vi "CE Measure.vi"(11 "CEmeter settings":T7={"AC Source"={"AC Source type"=enum."Fluke 5XXX calibrator", "VISA"="", "Ref. clock (Hz)"=0.0, "status ref"=refnum}, "TWM pipe"="\\\\.\\pipe\\TWM:server", "Measurement status ref"=refnum, "TWM Status ref"=refnum, "Abort ref"=refnum, "DC meter"={"DC meter type"=enum."H/A/K 3458", "DC meter VISA"="", "NPLC"=10, "status ref"=refnum}, "Measurement properties"={"Measurement frequencies (Hz)"=[1000.0], "Sampling frequency (Hz)"=500000.0, "Signal amplitude (V)"=4.5, "AC-DC settle time (s)"=20.0, "Record length (multiples of period)"=[1000.0, 10000.0, 1000.0], "Measurement template file"=path "", "Row of START keyword"=1, "Row of STOP keyword"=0, "Calculate RMS from samples"=FALSE, "AC-DC warm up time (s)"=300.0, "Measurement template line"=[], "DC meter readings No."=10, "Algorithm"="TWM-WFFT"}, "Skip waiting ref"=refnum, "Octave paths"={"GNU Octave path"=path "C:/Program Files/GNU Octave/Octave-6.2.0/mingw64/bin", "TWM+QWTB path"=path "C:/Users/labina/Desktop/TWM-1.8.7.0-full/octprog", "lvlib path"=path "D:/martin/WAC/WACsw - github/control_software/Filter function meter/external libraries/GOLPI 0.7.3.1 source distribution LV 20.0 32 bit/lv_proc.dll"}, "Template definition"={"Keywords column"=0, "Sig. freq. column"=1, "Rec. len. column"=2, "Meas. points. row min to read"=9, "Meas. points. row max to read"=1509, "Properties column"=4, "Properties row start"=1, "Properties row end"=5, "Keyword START regexp"="", "Keyword STOP regexp"="", "HW data column"=7, "HW data row start"=1, "HW data row end"=3, "TIme and date column start"=3, "Digitizer value column start "=4, "DC mean column start "=6, "DC readings column start"=10}} {"Measurement properties"."Record length (multiples of period)" format="%#_3p"; "Measurement properties"."Sampling frequency (Hz)" format="%#_3p"; "Measurement properties"."Measurement frequencies (Hz)" format="%#_3p"}) -> (0 "error out":errorcluster)   [LabVIEW 2020]
uses:
  external libraries/varilib/varilib.lvlib
  external libraries/TWM-1.8.7.0-client/TWM Client.lvlib
  <vilib>/Utility/error.llb/DialogType.ctl
  Utilities/Type definitions/Sampling properties.ctl
  <vilib>/Utility/NIReport.llb/NI_report.lvclass
  General AC source/Type definitions/AC Source.ctl
  General AC source/Type definitions/AC Source type.ctl
  General DC meter/Type definitions/DC meter.ctl
  General DC meter/Type definitions/DC meter type.ctl
  FR Measurement/Type definitions/FR Measuement properties.ctl
  FR Utilities/Type definitions/FR Template definition.ctl
panel:
  out "TWM result as string for XCL":string[][][](array[string])
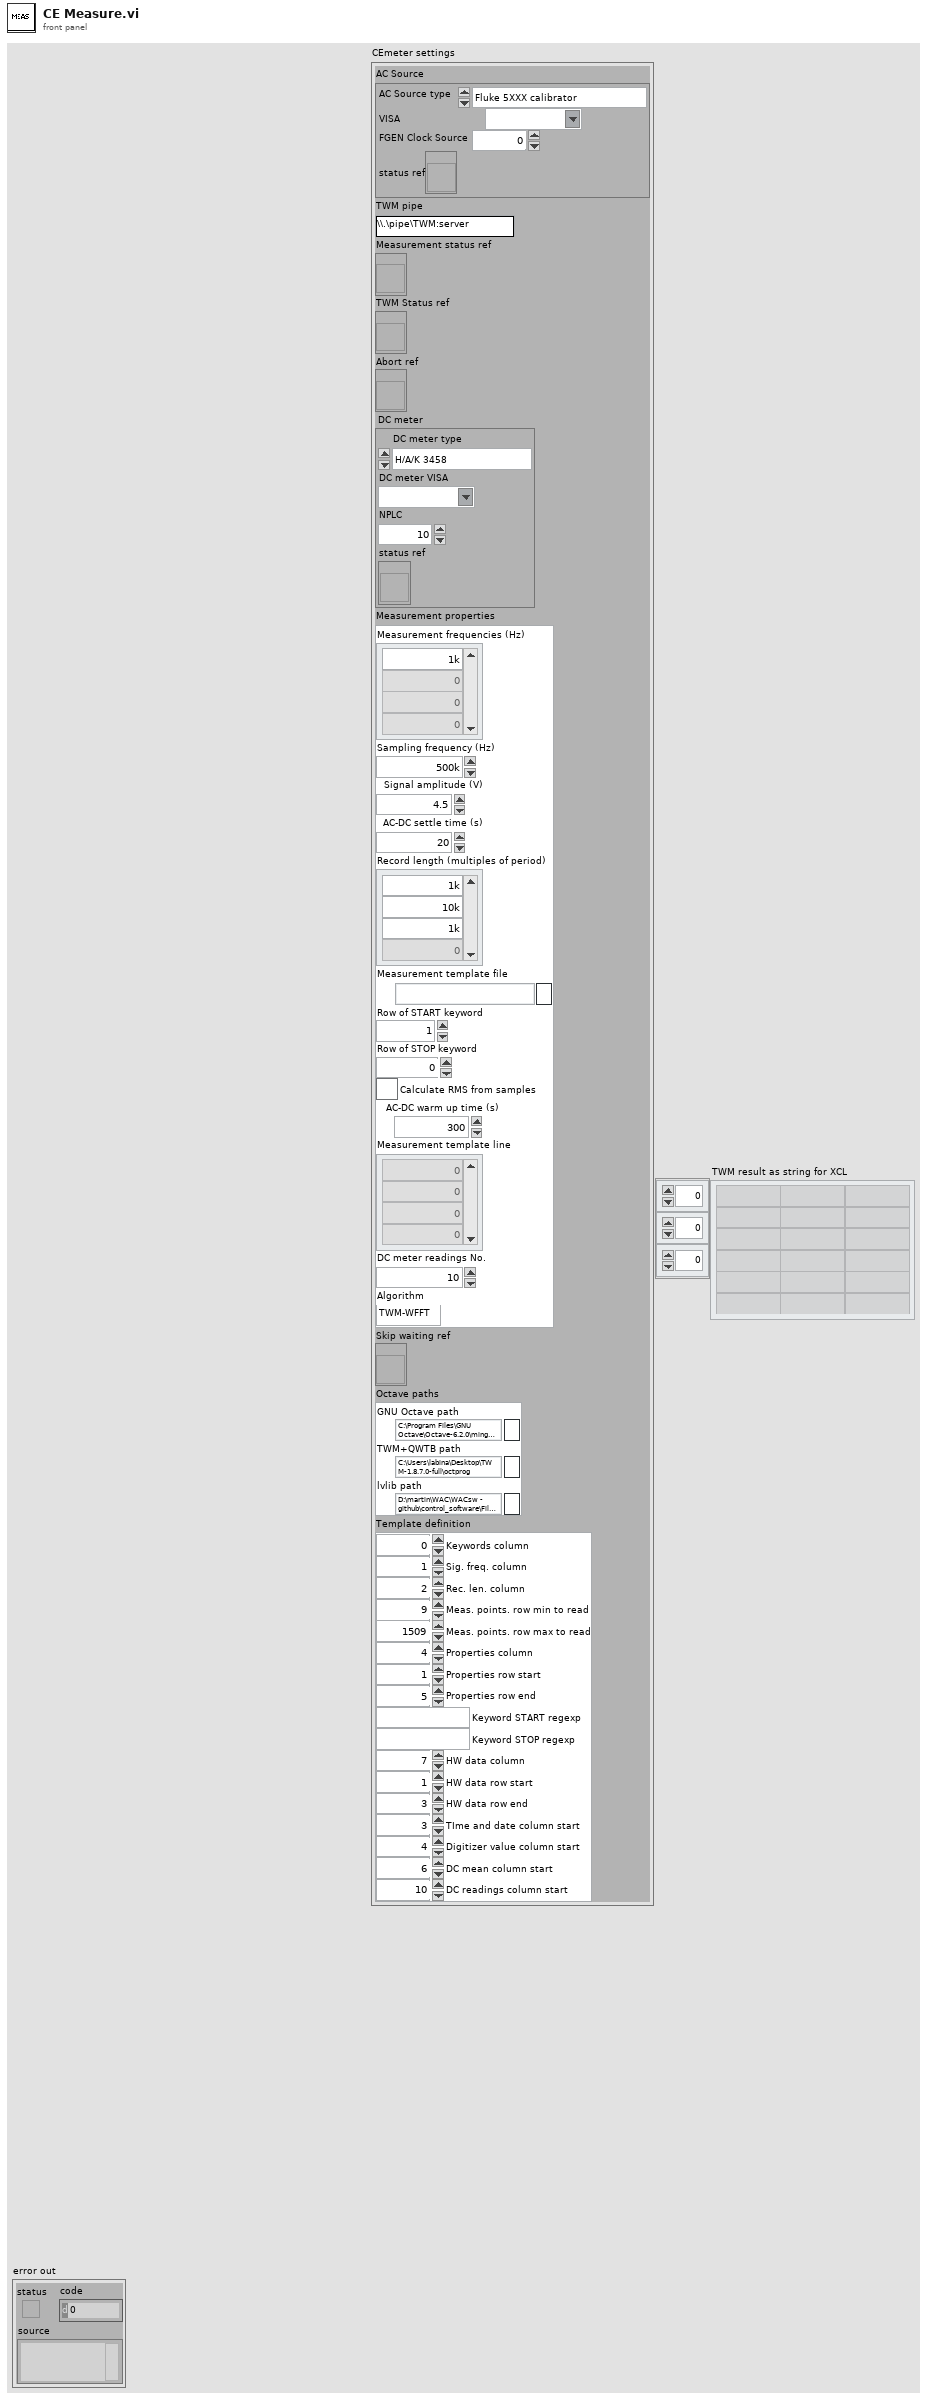
[diagram p1: front panel]
types:
  T1 = typedef "AC Source.ctl" = cluster{"AC Source type":T2, "VISA":refnum<visa-resource-name>, "Ref. clock (Hz)":dbl, "status ref":refnum<vi>}
  T2 = typedef "AC Source type.ctl" = enum16{"Fluke 5XXX calibrator", "Tektronix AFG3000 series", "dummy"}
  T3 = typedef "DC meter.ctl" = cluster{"DC meter type":T4, "DC meter VISA":refnum<visa-resource-name>, "NPLC":i32, "status ref":refnum<vi>}
  T4 = typedef "DC meter type.ctl" = enum16{"H/A/K 3458", "FLuke 8508A", "dummy"}
  T5 = typedef "FR Measuement properties.ctl" = cluster{"Measurement frequencies (Hz)":dbl[], "Sampling frequency (Hz)":dbl, "Signal amplitude (V)":dbl, "AC-DC settle time (s)":dbl, "Record length (multiples of period)":dbl[], "Measurement template file":path, "Row of START keyword":i32, "Row of STOP keyword":i32, "Calculate RMS from samples":bool, "AC-DC warm up time (s)":dbl, "Measurement template line":i32[], "DC meter readings No.":i32, "Algorithm":string}
  T6 = typedef "FR Template definition.ctl" = cluster{"Keywords column":i32, "Sig. freq. column":i32, "Rec. len. column":i32, "Meas. points. row min to read":i32, "Meas. points. row max to read":i32, "Properties column":i32, "Properties row start":i32, "Properties row end":i32, "Keyword START regexp":string, "Keyword STOP regexp":string, "HW data column":i32, "HW data row start":i32, "HW data row end":i32, "TIme and date column start":i32, "Digitizer value column start ":i32, "DC mean column start ":i32, "DC readings column start":i32}
  T7 = cluster{"AC Source":T1, "TWM pipe":string, "Measurement status ref":refnum<vi>, "TWM Status ref":refnum<vi>, "Abort ref":refnum<vi>, "DC meter":T3, "Measurement properties":T5, "Skip waiting ref":refnum<vi>, "Octave paths":cluster{"GNU Octave path":path, "TWM+QWTB path":path, "lvlib path":path}, "Template definition":T6}
  T8 = typedef "DialogType.ctl" = u16
  T9 = typedef "FFmeter settings.ctl" = cluster{"AC Source":T1, "TWM pipe":string, "Measurement status ref":refnum<vi>, "TWM Status ref":refnum<vi>, "Abort ref":refnum<vi>, "DC meter":T3, "Measurement properties":T5, "Skip waiting ref":refnum<vi>, "Octave paths":cluster{"GNU Octave path":path, "TWM+QWTB path":path, "lvlib path":path}, "Template definition":T6}
  T10 = typedef "Sampling properties.ctl" = cluster{"Sampling frequency (Hz)":dbl, "Record length (multiples of period)":dbl, "Signal amplitude (V)":dbl, "Measurement frequency (Hz)":dbl, "Calculate RMS from samples":bool, "Algorithm":string, "Measurement path":string}
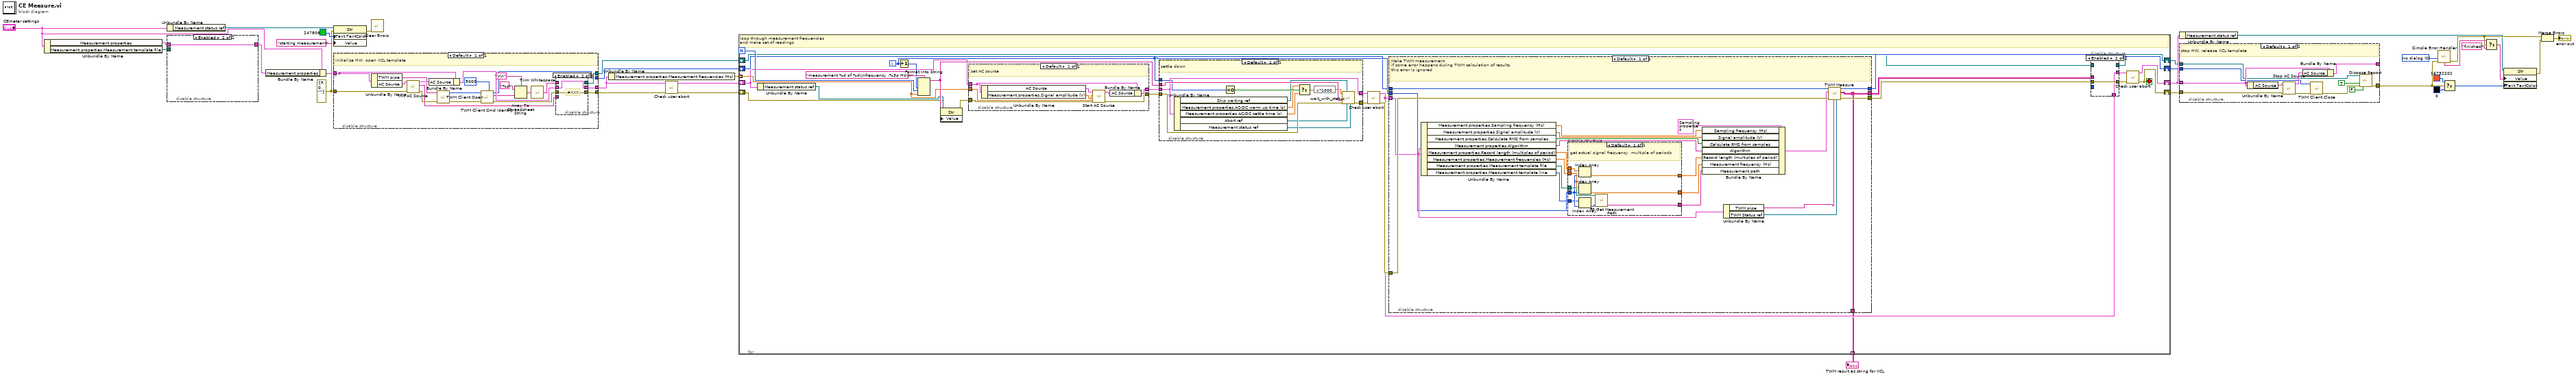
[diagram p0: block diagram]
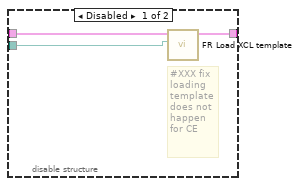
[diagram p2: hidden frame]
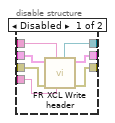
[diagram p3: hidden frame]
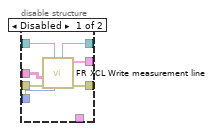
[diagram p4: hidden frame]
diagram:
  w30 = T8 0 items=["no dialog", "OK message", "continue or stop message", "OK message + warnings", "continue/stop + warnings"] ("type of dialog (OK msg:1)")
  w11 = errorcluster {"status"=FALSE, "code"=0, "source"=""} ("error out")
  n1 = Unbundle By Name("CEmeter settings") -> ("Measurement properties"=w9:T5, "Measurement properties.Measurement template file"=w5:path)
  n2 = Unbundle By Name("CEmeter settings") -> ("Measurement status ref"=w22:refnum<vi>)
  n3 = disable-structure shown="Enabled" {
    disable-tunnel: w9 -> [w37 w38]
    disable-tunnel: [w36 w38] -> w8
    disable-tunnel: w5 -> [w35 _]
    frame Disabled {
      # "#XXX fix\nloading\ntemplate\ndoes not\nhappen\nfor CE"
      n4 = call "FR Load XCL template.vi"("Measurement template file"=w35, "Measurement properties"=w37) -> ("Measurement properties out"=w36:T5)  [unwired: 9 in]
    }
    frame Enabled {
    }
  }
  n5 = Bundle By Name(cluster="CEmeter settings", "Measurement properties"=w8) -> (w6:T7)
  n6 = property class="Str"(reference=w22, error in=w11, "Text.TextColor"=u32 247808 ("Text.Text Colors:Text Color"), "Value"="starting measurement") -> (error out=w21:errorcluster)  [unwired: 1 out]
  n7 = disable-structure shown="Default" {
    disable-tunnel: w6 -> [w58]
    disable-tunnel: [w51] -> w2
    disable-tunnel: w11 -> [w56]
    disable-tunnel: [w54] -> w3
    disable-tunnel: [w43] -> w4
    disable-tunnel: [w52] -> w13
    frame Enabled {
      # "initialize HW, open XCL template"
      n8 = Unbundle By Name(w58) -> ("TWM pipe"=w55:string, "AC Source"=w59:T1)
      n9 = call "Init AC Source.vi"("error in (no error)"=w56, "AC source"=w59) -> ("error out"=w39:errorcluster, "Init status"=w50:string, "AC source out"=w57:T1)  [unwired: 7 in]
      n10 = Bundle By Name(cluster=w58, "AC Source"=w57) -> (w53:T7)
      n11 = call "TWM Client Open.vi"("error in"=w39, "pipe name"=w55) -> ("error out"=w45:errorcluster, "handle out"=w46:i32)  [unwired: 8 in]
      n12 = call "TWM Client Cmd Identify.vi"("timeout [ms]"=5000, "error in"=w45, "handle"=w46) -> ("error out"=w44:errorcluster, "channel idns"=w49:string[], "handle out"=w43:i32)  [unwired: 5 in, 1 out]
      n13 = Array To Spreadsheet String(delimiter (Tab)="\r\n", array=w49, 3:"%s" ("format string")) -> (spreadsheet string=w42:string)
      n14 = call <vilib>:"Trim Whitespace.vi"("string"=w42) -> ("trimmed string"=w41:string)  [unwired: 1 in]
      n15 = disable-structure shown="Enabled" {
        disable-tunnel: [w66 w67] -> w54
        disable-tunnel: w53 -> [w65 w68]
        disable-tunnel: [w64 _] -> w52
        disable-tunnel: [w63 w68] -> w51
        disable-tunnel: w50 -> [w62 _]
        disable-tunnel: w44 -> [w61 w67]
        disable-tunnel: w41 -> [w60 _]
        frame Disabled {
          n16 = call "FR XCL Write header.vi"("AC source idn"=w62, "Digitizer idn"=w60, "error in (no error)"=w61, "FFmeter settings"=w65) -> ("error out"=w66:errorcluster, "FFmeter settings out"=w63:T9, "NI_report out"=w64:refnum<class "NI_report.lvclass">)  [unwired: 5 in]
        }
        frame Enabled {
          # "#XXX"
        }
      }
    }
  }
  n17 = call <vilib>:"Clear Errors.vi"("error in (no error)"=w21) -> ()  [unwired: 5 in, 2 out]
  n18 = Unbundle By Name(w2) -> ("Measurement properties.Measurement frequencies (Hz)"=w34:dbl[])
  n19 = call "Check user abort.vi"("error in (no error)"=w3, "FFmeter settings"=w2) -> ("error out"=w20:errorcluster, "FFmeter settings out"=w19:T9)  [unwired: 8 in]
  n20 = for {
    N -> [w92]
    shift-right: [w82] -> w17
    shift-left: w20 -> [w86]
    shift-right: [w81] -> w15
    shift-left: w19 -> [w73]
    tunnel: w34 -> [w87] mode=indexing
    shift-right: [w77] -> w12
    shift-left: w13 -> [w76]
    shift-right: [w80] -> w14
    shift-left: w4 -> [w74]
    tunnel: [w69] -> w1 mode=indexing
    i -> [w72]
    stop <- w82 stop-if-true
    # "loop through measurement frequencies\nand make set of readings"
    n21 = Unbundle By Name(w73) -> ("Measurement status ref"=w91:refnum<vi>)
    n22 = Increment(x=w72) -> (x+1=w93:i32)
    n23 = Format Into String(format string="measurement %d of %d\\nfrequency :%3p Hz\\n", w93, w92, w87) -> (resulting string=w94:string)  [unwired: 2 in, 1 out]
    n24 = property class="Str"(reference=w91, error in=w86, "Value"=w94) -> (error out=w90:errorcluster)  [unwired: 1 out]
    n25 = disable-structure shown="Default" {
      disable-tunnel: w73 -> [w124]
      disable-tunnel: w90 -> [w123]
      disable-tunnel: [w122] -> w89
      disable-tunnel: [w125] -> w88
      disable-tunnel: w87 -> [w119]
      frame Enabled {
        # "set AC source"
        n26 = Unbundle By Name(w124) -> ("AC Source"=w120:T1, "Measurement properties.Signal amplitude (V)"=w118:dbl)
        n27 = call "Start AC Source.vi"("error in (no error)"=w123, "Signal amplitude (V)"=w118, "Signal frequency  (Hz)"=w119, "AC source"=w120) -> ("error out"=w122:errorcluster, "AC source out"=w121:T1)  [unwired: 5 in, 1 out]
        n28 = Bundle By Name(cluster=w124, "AC Source"=w121) -> (w125:T9)
      }
    }
    n29 = disable-structure shown="Default" {
      disable-tunnel: w94 -> [w117]
      disable-tunnel: [w111] -> w85
      disable-tunnel: [w115] -> w83
      disable-tunnel: w89 -> [w116]
      disable-tunnel: w88 -> [w115]
      disable-tunnel: w72 -> [w110]
      frame Enabled {
        # "settle down"
        n30 = Unbundle By Name(w115) -> ("Skip waiting ref"=w105:refnum<vi>, "Measurement properties.AC-DC warm up time (s)"=w108:dbl, "Measurement properties.AC-DC settle time (s)"=w107:dbl, "Abort ref"=w113:refnum<vi>, "Measurement status ref"=w112:refnum<vi>)
        n31 = Equal To 0?(x=w110) -> (x = 0?=w109:bool)
        n32 = Select(t=w108, s=w109, f=w107) -> (s? t:f=w106:dbl)
        n33 = expression code="x*1000"(w106) -> (w114:dbl)
        n34 = call "wait_with_status.vi"("stat ref"=w112, "stop ref"=w113, "second stop ref"=w105, "error in"=w116, "comment"=w117, "ms to wait"=w114) -> ("error out"=w111:errorcluster)  [unwired: 4 in, 1 out]
      }
    }
    n35 = call "Check user abort.vi"("error in (no error)"=w85, "FFmeter settings"=w83) -> ("error out"=w84:errorcluster, "FFmeter settings out"=w70:T9)  [unwired: 8 in]
    n36 = disable-structure shown="Default" {
      disable-tunnel: [w146] -> w71
      disable-tunnel: w84 -> [w147]
      disable-tunnel: w70 -> [w130]
      disable-tunnel: w74 -> [w126]
      disable-tunnel: [w145] -> w80
      disable-tunnel: w72 -> [w144]
      disable-tunnel: [w143] -> w75
      disable-tunnel: [w143] -> w69
      frame Enabled {
        # "Make TWM measurement\nif some error happens during TWM calculation of results,\nthis error is ignored"
        n37 = Unbundle By Name(w130) -> ("Measurement properties.Sampling frequency (Hz)"=w132:dbl, "Measurement properties.Signal amplitude (V)"=w138:dbl, "Measurement properties.Calculate RMS from samples"=w139:bool, "Measurement properties.Algorithm"=w140:string, "Measurement properties.Record length (multiples of period)"=w133:dbl[], "Measurement properties.Measurement frequencies (Hz)"=w134:dbl[], "Measurement properties.Measurement template file"=w141:path, "Measurement properties.Measurement template line"=w142:i32[])
        n38 = disable-structure shown="Default" {
          disable-tunnel: w134 -> [w156]
          disable-tunnel: w133 -> [w155]
          disable-tunnel: w126 -> [w152]
          disable-tunnel: [w154] -> w137
          disable-tunnel: w141 -> [w153]
          disable-tunnel: w142 -> [w151]
          disable-tunnel: [w149] -> w135
          disable-tunnel: [w148] -> w136
          frame Enabled {
            # "get actual signal frequency, multiple of periods"
            n39 = Index Array(array=w155, index=w152) -> (element=w148:dbl)
            n40 = Index Array(array=w156, index=w152) -> (element=w149:dbl)
            n41 = Index Array(array=w151, index=w152) -> (element=w150:i32)
            n42 = call "FR Get Measurement Path.vi"("Template line"=w150, "Measurement template file"=w153) -> ("Measurement path as string"=w154:string)  [unwired: 8 in, 1 out]
          }
        }
        n43 = Bundle By Name(cluster=T10 {"Sampling frequency (Hz)"=500000.0, "Record length (multiples of period)"=1000.0, "Signal amplitude (V)"=4.5, "Measurement frequency (Hz)"=1000.0, "Calculate RMS from samples"=FALSE, "Algorithm"="TWM-WFFT", "Measurement path"=""} ("TWM Measurement properties"), "Sampling frequency (Hz)"=w132, "Signal amplitude (V)"=w138, "Calculate RMS from samples"=w139, "Algorithm"=w140, "Record length (multiples of period)"=w136, "Measurement frequency (Hz)"=w135, "Measurement path"=w137) -> (w127:T10)
        n44 = Unbundle By Name(w130) -> ("TWM pipe"=w129:string, "TWM Status ref"=w128:refnum<vi>)
        n45 = call "TWM Measure.vi"("TWM Status ref"=w128, "TWM pipe"=w129, "error in (no error)"=w147, "TWM Measurement properties"=w127, "TWM handle"=w144) -> ("error out"=w146:errorcluster, "TWM result as string"=w143:string[][], "TWM handle out"=w145:i32)  [unwired: 4 in]
      }
    }
    n46 = disable-structure shown="Enabled" {
      disable-tunnel: [w102 w104] -> w79
      disable-tunnel: [w101 w103] -> w78
      disable-tunnel: [w100 _] -> w77
      disable-tunnel: w76 -> [w99 _]
      disable-tunnel: w75 -> [w98 _]
      disable-tunnel: _ -> [w97 _]
      disable-tunnel: w71 -> [w96 w104]
      disable-tunnel: w70 -> [_ w103]
      frame Disabled {
        n47 = call "FR XCL Write measurement line.vi"("Iteration index"=w97, "report in"=w99, "error in (no error)"=w96, "TWM result as string for XCL"=w98) -> ("error out"=w102:errorcluster, "FFmeter settings out"=w101:T9, "report out"=w100:refnum<class "NI_report.lvclass">)  [unwired: 5 in]
      }
      frame Enabled {
      }
    }
    n48 = call "Check user abort.vi"("error in (no error)"=w79, "FFmeter settings"=w78) -> ("error out"=w82:errorcluster, "FFmeter settings out"=w81:T9)  [unwired: 8 in]
  }
  "TWM result as string for XCL" <- w1
  n49 = Unbundle By Name(w15) -> ("Measurement status ref"=w18:refnum<vi>)
  n50 = disable-structure shown="Default" {
    disable-tunnel: w15 -> [w168]
    disable-tunnel: [w167] -> _
    disable-tunnel: [w161] -> w16
    disable-tunnel: w17 -> [w164]
    disable-tunnel: w14 -> [w163]
    disable-tunnel: w12 -> [w160]
    frame Enabled {
      # "stop HW, release XCL template"
      n51 = Unbundle By Name(w168) -> ("AC Source"=w166:T1)
      n52 = call "Stop AC Source.vi"("error in (no error)"=w164, "AC source"=w166) -> ("error out"=w157:errorcluster, "AC source out"=w165:T1)  [unwired: 8 in]
      n53 = Bundle By Name(cluster=w168, "AC Source"=w165) -> (w167:T9)
      n54 = call "TWM Client Close.vi"("error in"=w157, "handle in"=w163) -> ("error out"=w162:errorcluster)  [unwired: 9 in]
      n55 = call-dynamic "Dispose Report.vi"("report in"=w160, "save changes? (F)"=TRUE, "error in (no error)"=w162, "close report? (T)"=FALSE) -> ("error out"=w161:errorcluster)  [unwired: 11 in]
    }
  }
  n56 = call <vilib>:"Simple Error Handler.vi"("type of dialog (OK msg:1)"=w30, "error in (no error)"=w16) -> ("error out"=w25:errorcluster, "message"=w33:string)  [unwired: 3 in, 3 out]
  n57 = Select(t=u32 16732202 ("Text.Text Colors:Text Color"), s=w16, f=u32 0 ("Text.Text Colors:Text Color")) -> (s? t:f=w27:u32)
  n58 = Select(t=w33, s=w25, f="finished") -> (s? t:f=w31:string)
  n59 = property class="Str"(reference=w18, "Value"=w31, "Text.TextColor"=w27) -> (error out=w26:errorcluster)  [unwired: 1 in, 1 out]
  n60 = Merge Errors(w25, w26) -> (→"error out":errorcluster)
